vi "BeltDrive.vi"(0 "button9":bool, 2 "shootSpeedValueBot":dbl, 4 "encoderBottomFeedback":dbl, 5 "shootSpeedValueTop":dbl, 6 "encoderTopFeedback":dbl, 7 "percent":dbl, 8 "botLimit":bool, 9 "midLimit":bool, 10 "topLimit":bool, 11 "shootButton":bool) -> (1 "botMotor":i8, 3 "topMotor":i8)   [LabVIEW 2011]
uses:
  Robot Global Data.vi
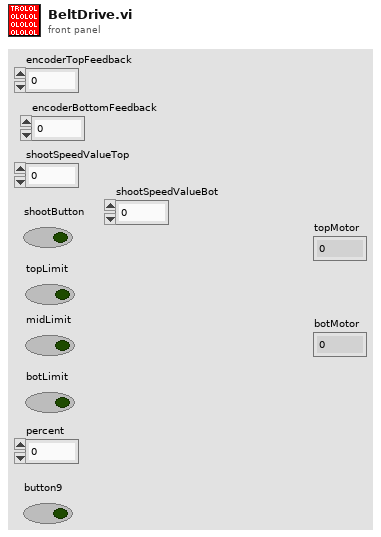
[diagram p1: front panel]
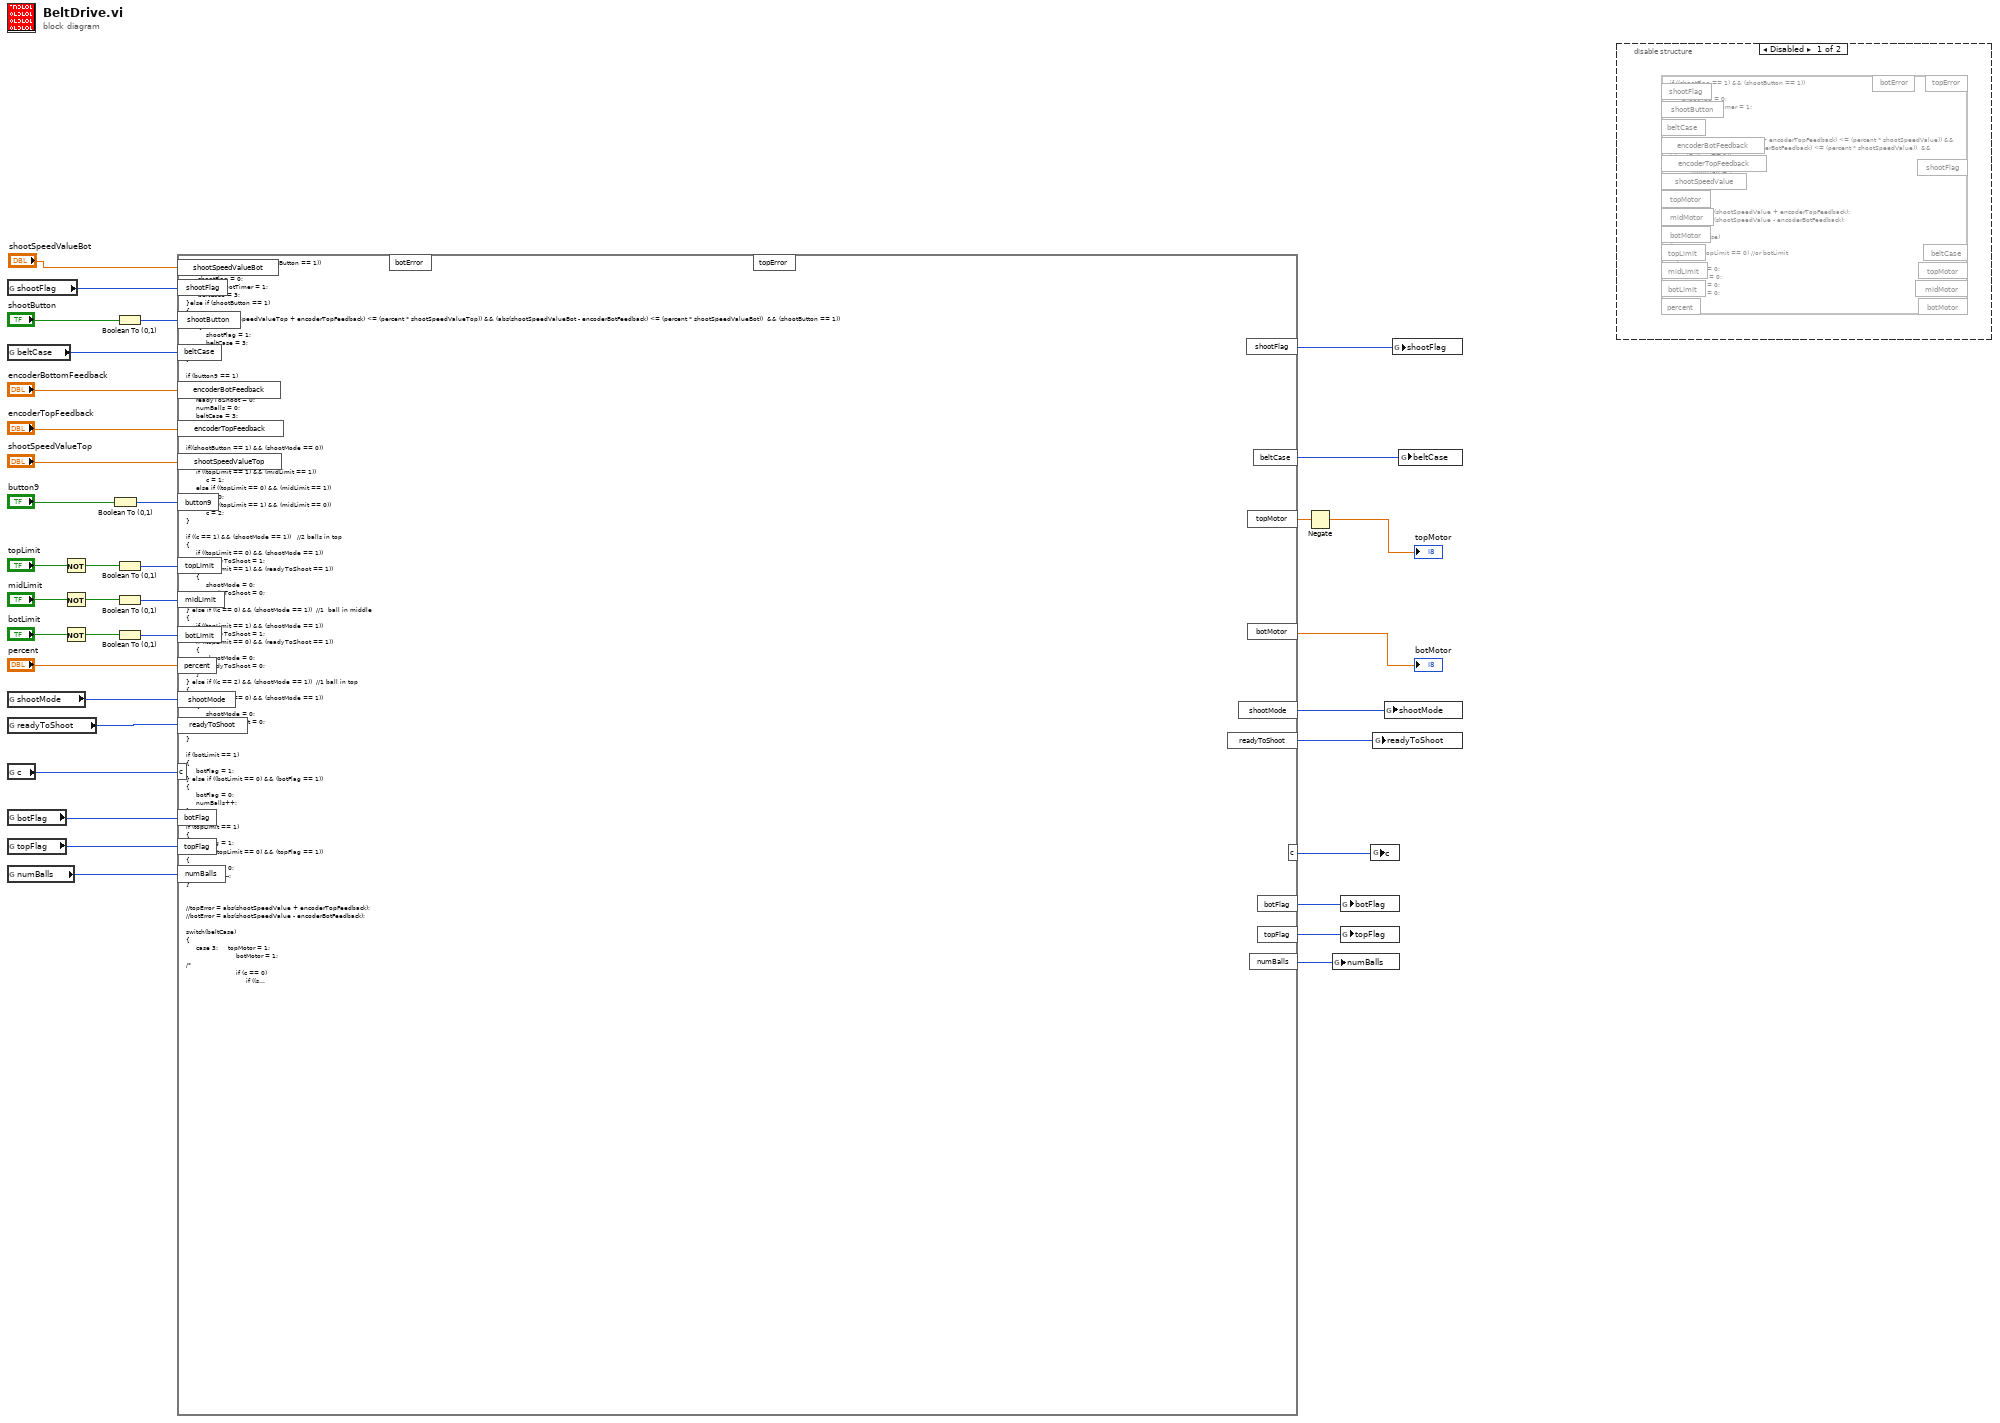
[diagram p0: block diagram]
diagram:
  n1 = global read "Robot Global Data.vi" "shootFlag"() -> (w37:u8)
  n2 = global read "Robot Global Data.vi" "beltCase"() -> (w36:i8)
  n3 = global read "Robot Global Data.vi" "shootMode"() -> (w20:u8)
  n4 = global read "Robot Global Data.vi" "readyToShoot"() -> (w18:u8)
  n5 = global read "Robot Global Data.vi" "c"() -> (w14:i8)
  n6 = global read "Robot Global Data.vi" "botFlag"() -> (w12:i8)
  n7 = global read "Robot Global Data.vi" "topFlag"() -> (w11:i8)
  n8 = global read "Robot Global Data.vi" "numBalls"() -> (w10:i8)
  n9 = Not(x="topLimit") -> (.not. x?=w30:bool)
  n10 = Not(x="midLimit") -> (.not. x?=w29:bool)
  n11 = Not(x="botLimit") -> (.not. x?=w28:bool)
  n12 = Boolean To (0,1)(Boolean="button9") -> (0, 1=w3:i16)
  n13 = Boolean To (0,1)(Boolean="shootButton") -> (0, 1=w34:i16)
  n14 = Boolean To (0,1)(Boolean=w30) -> (0, 1=w6:i16)
  n15 = Boolean To (0,1)(Boolean=w29) -> (0, 1=w5:i16)
  n16 = Boolean To (0,1)(Boolean=w28) -> (0, 1=w4:i16)
  n17 = formula code="if ((shootFlag == 1) && (shootButton == 1))\n{\n\t     shootFlag = 0;\n\t     //resetShootTimer = 1;\n\t     beltCase = 3;\n}else if (shootButton == 1)\n{\n\t     if ((abs(shootSpeedValueTop + encoderTopFeedback) <= (percent * shootSpeedValueTop)) && (abs(shootSpeedValueBot - encoderBotFeedback) <= (percent * shootSpeedValueBot))  && (shootButton == 1))\n\t     {\n\t\t        shootFlag = 1;\n          beltCase = 3;\n     \t}\n}\n\nif (button9 == 1)\n{\n     shootMode = 0;\n     readyToShoot = 0;\n     numBalls = 0;\n     beltCase = 3;\n}\n\n\nif((shootButton == 1) && (shootMode == 0))\n{\n     shootMode = 1;\n     if ((topLimit == 1) && (midLimit == 1))\n          c = 1;\n     else if ((topLimit == 0) && (midLimit == 1))\n          c = 0;\n     else if ((topLimit == 1) && (midLimit == 0))\n          c = 2;\n}\n\nif ((c == 1) && (shootMode == 1))   //2 balls in top\n{\n     if ((topLimit == 0) && (shootMode == 1))  \n          readyToShoot = 1;\n     if ((topLimit == 1) && (readyToShoot == 1)) \n     {\n          shootMode = 0;\n          readyToShoot = 0;\n     }\n} else if ((c == 0) && (shootMode == 1))  //1  ball in middle\n{\n     if ((topLimit == 1) && (shootMode == 1))  \n          readyToShoot = 1;\n     if ((topLimit == 0) && (readyToShoot == 1))  \n     {\n          shootMode = 0;\n          readyToShoot = 0;\n     }\n} else if ((c == 2) && (shootMode == 1))  //1 ball in top\n{\n     if ((topLimit == 0) && (shootMode == 1))  \n     {\n          shootMode = 0;\n          readyToShoot = 0;\n     }\n}\n\nif (botLimit == 1)\n{\n     botFlag = 1;\n} else if ((botLimit == 0) && (botFlag == 1))\n{\n     botFlag = 0;\n     numBalls++;\n}\n\nif (topLimit == 1)\n{\n     topFlag = 1;\n} else if ((topLimit == 0) && (topFlag == 1))\n{\n     topFlag = 0;\n     numBalls--;\n}     \n\n\n//topError = abs(shootSpeedValue + encoderTopFeedback);\n//botError = abs(shootSpeedValue - encoderBotFeedback);\n\nswitch(beltCase)\n{\n     case 3:     topMotor = 1;\n                         botMotor = 1;\n/*\n                         if (c == 0)\n                              if ((shootMode == 0) && ((topLimit == 1) && (botLimit == 0)))\n                                   beltCase = 2;\n                         else\n                              if ((shootMode == 0) && ((topLimit == 1) && (midLimit == 1) && (botLimit == 0)))\n                                   beltCase = 2;\n*/\n                         //if ( (shootMode == 0) && (((topLimit == 0) && (midLimit == 1) && (botLimit == 0)) || ((topLimit == 1) && (botLimit == 0))))\n                         //if ((shootMode == 0) && ((topLimit == 1) && (botLimit == 0)))\n                         if (numBalls == 1)\n                         {\n                              //if ((shootMode == 0) && ((midLimit == 1) && (botLimit == 0)))\n                              if ( (shootMode == 0) && (((topLimit == 0) && (midLimit == 1) && (botLimit == 0)) || ((topLimit == 1) && (botLimit == 0))))\n                              {\n                                   beltCase = 2;\n                              }\n                         } else if (numBalls >= 2)\n                         {\n                              if ((shootMode == 0) && ((topLimit == 1) && (midLimit == 1) && (botLimit == 0)))\n                              {\n                                   beltCase = 2;\n                              }\n                         }\n                              //beltCase = 2;\n                         break;\n     case 2:     topMotor = 0;\n                         botMotor = 1;\n                         if ((shootButton == 1))\n                              beltCase = 3;\n                         else if (botLimit == 1)\n                              if (topLimit == 1)\n                                   beltCase = 0;\n                              else if ((topLimit == 0) && (midLimit == 1))\n                                   beltCase = 3;\n                         break;\n     default:     topMotor = 0;\n                         botMotor = 0;\n                         if (shootButton == 1)\n                              beltCase = 3;\n                         break;\n}"("shootFlag"=w37, "shootButton"=w34, "beltCase"=w36, "topLimit"=w6, "midLimit"=w5, "botLimit"=w4, "encoderTopFeedback"="encoderTopFeedback", "shootSpeedValueTop"="shootSpeedValueTop", "percent"="percent", "encoderBotFeedback"="encoderBottomFeedback", "shootMode"=w20, "readyToShoot"=w18, "c"=w14, "botFlag"=w12, "topFlag"=w11, "numBalls"=w10, "button9"=w3, "shootSpeedValueBot"="shootSpeedValueBot") -> ("shootFlag"=w35:u8, "beltCase"=w16:i8, "topMotor"=w24:dbl, "botMotor"=→"botMotor":dbl, "shootMode"=w19:u8, "readyToShoot"=w17:u8, "c"=w13:i8, "botFlag"=w9:i8, "topFlag"=w8:i8, "numBalls"=w7:i8)  [unwired: 2 out]
  n18 = Negate(x=w24) -> (-x=→"topMotor":dbl)
  n19 = global write "Robot Global Data.vi" "numBalls"(w7) -> ()
  n20 = global write "Robot Global Data.vi" "botFlag"(w9) -> ()
  n21 = global write "Robot Global Data.vi" "topFlag"(w8) -> ()
  n22 = global write "Robot Global Data.vi" "c"(w13) -> ()
  n23 = global write "Robot Global Data.vi" "readyToShoot"(w17) -> ()
  n24 = global write "Robot Global Data.vi" "shootMode"(w19) -> ()
  n25 = global write "Robot Global Data.vi" "shootFlag"(w35) -> ()
  n26 = global write "Robot Global Data.vi" "beltCase"(w16) -> ()
  n27 = disable-structure shown="Disabled" {
    frame Disabled {
      n28 = formula code="if ((shootFlag == 1) && (shootButton == 1))\n{\n\t     shootFlag = 0;\n\t     //resetShootTimer = 1;\n\t     beltCase = 4;\n}else\n{\n\t     if ((abs(shootSpeedValue + encoderTopFeedback) <= (percent * shootSpeedValue)) && (abs(shootSpeedValue - encoderBotFeedback) <= (percent * shootSpeedValue))  && (shootButton == 1))\n\t     {\n\t\t        shootFlag = 1;\n          beltCase = 4;\n     \t}\n}\n\ntopError = abs(shootSpeedValue + encoderTopFeedback);\nbotError = abs(shootSpeedValue - encoderBotFeedback);\n\nswitch(beltCase)\n{\n\tcase 4:\tif (topLimit == 0) //or botLimit\n\t\t\t{\n\t\t\t\ttopMotor = 0;\n\t\t\t\tmidMotor = 0;\n\t\t\t\tbotMotor = 0;\n\t\t\t\tbeltCase = 0;\n\t\t\t} else\n\t\t\t{\n\t\t\t\ttopMotor = 1;\n\t\t\t\tmidMotor = 1;\n\t\t\t\tbotMotor = 1;\n\t\t\t}\n\t\t\tbreak;\n\t\t\t\t\n\tcase 3:\ttopMotor = 1;\n\t\t\tmidMotor = 1;\n\t\t\tbotMotor = 1;\n\t\t\tif (topLimit == 1)\n\t\t\t\tbeltCase = 0;\n\t\t\tbreak;\n\t\n\tcase 2:\ttopMotor = 0;\n\t\t\tmidMotor = 1;\n\t\t\tbotMotor = 1;\n\t\t\tif (midLimit == 1)\n\t\t\t\tbeltCase = 0;\n\t\t\tbreak;\n\t\t\t\n\tcase 1:\ttopMotor = 0;\n\t\t\tmidMotor = 0;\n\t\t\tbotMotor = 1;\n\t\t\tif (botLimit == 1)\n\t\t\t\tbeltCase = 0;\n\t\t\tbreak;\n\t\t\t\n\tdefault:\n\t\t\ttopMotor = 0;\n\t\t\tmidMotor = 0;\n\t\t\tbotMotor = 0;\n\t\t\t\n\t\t\tif (topLimit == 0)\n\t\t\t\tbeltCase = 3;\n\t\t\telse if (midLimit == 0)\n\t\t\t\tbeltCase = 2;\n\t\t\telse if (botLimit == 0)\n\t\t\t\tbeltCase = 1;\n\t\t\telse\n\t\t\t\tbeltCase = 0;\n\t\t\tbreak;\n\t\t\t\t\n}"() -> ()  [unwired: 13 in, 7 out]
    }
    frame Enabled {
    }
  }
